vi "LVClass_CameraSet ctor from Camera.vi"(0 "CameraSet (const)":refnum<class "CameraSet.lvclass">, 5 "Camera":refnum<class "Camera.lvclass">, 11 "error in (no error)":errorcluster) -> (4 "CameraSet (new)":refnum<class "CameraSet.lvclass">, 6 "Camera (dup)":refnum<class "Camera.lvclass">, 15 "error out":errorcluster)   [LabVIEW 2020, in "CameraSet.lvclass"]
doc: "CameraSet constructor from camera.\n\n<B>camera_setIn</B> : Constant Pointer to CameraSet object.\n<B>camera_setOut</B> : Constant Pointer to CameraSet object.\n<B>Camera</B> : Camera object."
uses:
  CameraSet.lvclass
  Camera.lvclass
  Handle creation.ctl
  CameraSet.lvclass/CameraSet.ctl
  LVClass_Camera read camera.vi
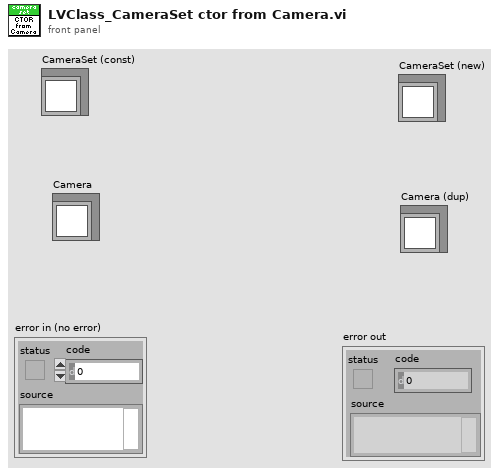
[diagram p1: front panel]
types:
  T1 = typedef "Handle creation.ctl" = enum16{"By ctor", "By write function"}
  T2 = typedef "ClassID.ctl" = i64
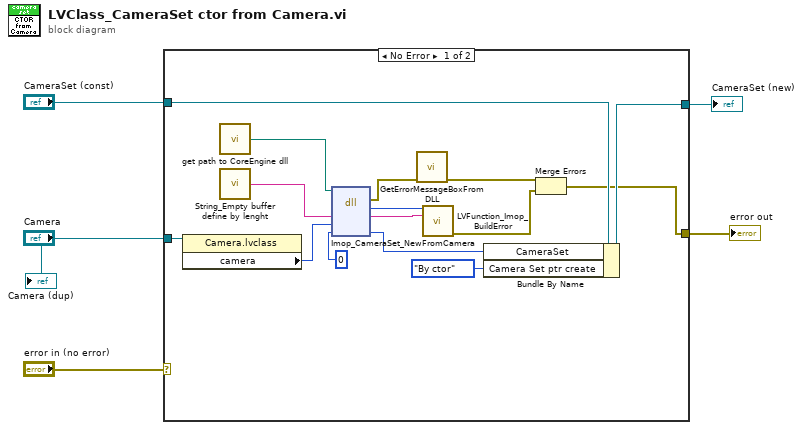
[diagram p0: block diagram]
diagram:
  n1 = case shown="No Error" "error in (no error)" {
    selector: "error in (no error)" -> [_ w21]
    tunnel: "Camera" -> [w7 _]
    tunnel: "CameraSet (const)" -> [w15 w22]
    tunnel: [w14 w22] -> w3
    tunnel: [w8 w21] -> w2
    frame No Error {
      n2 = property class="Camera.lvclass"(reference=w7) -> ("camera"=w6:T2)  [unwired: 1 in, 2 out]
      n3 = call "get path to CoreEngine dll.vi"() -> ("path to wavekit library"=w13:path)  [unwired: 14 in, 1 out]
      n4 = call "String_Empty buffer define by lenght.vi"() -> ("Empty buffer"=w20:string)  [unwired: 1 in]
      n5 = dll-call lib="D:/soft/HASO_v3/SVN_trunk/ImOpCoreEngine4_LV2011/DLLs/c_interface_vc100.dll" fn="Imop_CameraSet_NewFromCamera"(path in=w13, "message"=w20, "Camera"=w6, "objet"=0) -> (error out=w12:errorcluster, "return type"=w17:i32, "message"=w18:string, "objet"=w19:i64)  [unwired: 3 in, 1 out]
      n6 = call "GetErrorMessageBoxFromDLL.vi"("error IN"=w12) -> ("error OUT"=w10:errorcluster)  [unwired: 10 in]
      n7 = call "LVFunction_Imop_BuildError.vi"("code"=w17, "String to Prepend to source (\"\")"=w18) -> ("error out"=w9:errorcluster)  [unwired: 13 in]
      n8 = Bundle By Name(cluster=w15, "CameraSet"=w19, "Camera Set ptr create"=Handle_creation."By ctor") -> (w14:refnum<class "CameraSet.lvclass">)
      n9 = Merge Errors(w10, w9) -> (w8:errorcluster)
    }
    frame Error {
    }
  }
  "CameraSet (new)" <- w3
  "error out" <- w2
  "Camera (dup)" <- "Camera"
